vi "Read value (Boolean).vi"(8 "error in (no error)":errorcluster, 9 "default value":bool, 11 "JSON String in":refnum<class "JSON Boolean.lvclass">) -> (0 "error out":errorcluster, 2 "value":bool)   [LabVIEW 2015, in "LVJSON.lvlib" / "JSON Boolean.lvclass"]
uses:
  JSON Boolean.lvclass
  JSON Boolean.lvclass/JSON Boolean.ctl
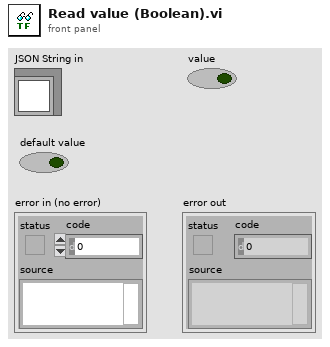
[diagram p1: front panel]
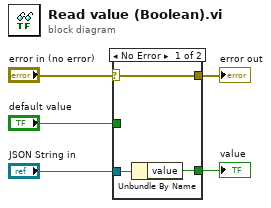
[diagram p0: block diagram]
diagram:
  n1 = case shown="No Error" "error in (no error)" {
    selector: "error in (no error)" -> [w8 w10]
    tunnel: [w8 w10] -> w4
    tunnel: "JSON String in" -> [w7 _]
    tunnel: [w6 w9] -> w2
    tunnel: "default value" -> [_ w9]
    frame No Error {
      n2 = Unbundle By Name(w7) -> ("value"=w6:bool)
    }
    frame Error {
    }
  }
  "error out" <- w4
  "value" <- w2
